vi "rsidr_core_global.vi"() -> ()   [LabVIEW 2020, in "Rohde&Schwarz CMWXP NR FR1 Measurement.lvlib"] (continued)
 "Rngtable Callback"="", "Coerce Callback"="", "Supported Models"="", "Instrument Options"="", "Check Status Callback"="", "Flags"=0, "Help"="Defines an upper limit for the carrier frequency error.\n\nAvailable Repeated Capabilities:\ninstance: i0, i1, i2, i3, i4, i5, i6, i7, i8, i9, i10, i11, i12, i13, i14, i15, i16, i17, i18, i19, i20, i21, i22, i23, i24, i25, i26, i27, i28, i29, i30, i31, i32\r\n\nRemote-control command(s):\nCONFigure:NRSub:MEAS<i>:PRACh:LIMit:FERRor"}, {"Level"=4, "Class Only"=FALSE, "Identifier"="RSCMWXPNRFR1M_ATTR_PRACH_LIMIT_FREQUENCY_ERROR_ENABLED", "Descriptive Name"="PRACH Limit Frequency Error Enabled", "Data Type"=enum."ViBoolean", "Command"="CONF:NRS:MEAS{instance}:PRAC:LIM:FERR", "Access"=enum."Read/Write", "Range Table"="", "Read Callback"="", "Write Callback"="", "Range Callback"="", "Check Callback"="", "Rngtable Callback"="", "Coerce Callback"="", "Supported Models"="", "Instrument Options"="", "Check Status Callback"="", "Flags"=0, "Help"="Enables or disables the limit check.\n\nAvailable Repeated Capabilities:\ninstance: i0, i1, i2, i3, i4, i5, i6, i7, i8, i9, i10, i11, i12, i13, i14, i15, i16, i17, i18, i19, i20, i21, i22, i23, i24, i25, i26, i27, i28, i29, i30, i31, i32\r\n\nRemote-control command(s):\nCONFigure:NRSub:MEAS<i>:PRACh:LIMit:FERRor"}, {"Level"=2, "Class Only"=TRUE, "Identifier"="", "Descriptive Name"="Results", "Data Type"=enum."ViInt32", "Command"="", "Access"=enum."Read Only", "Range Table"="", "Read Callback"="", "Write Callback"="", "Range Callback"="", "Check Callback"="", "Rngtable Callback"="", "Coerce Callback"="", "Supported Models"="", "Instrument Options"="", "Check Status Callback"="", "Flags"=0, "Help"="Results of the NR FR1 PRACH measurement"}, {"Level"=3, "Class Only"=TRUE, "Identifier"="", "Descriptive Name"="Detected Signal Configuration", "Data Type"=enum."ViInt32", "Command"="", "Access"=enum."Read Only", "Range Table"="", "Read Callback"="", "Write Callback"="", "Range Callback"="", "Check Callback"="", "Rngtable Callback"="", "Coerce Callback"="", "Supported Models"="", "Instrument Options"="", "Check Status Callback"="", "Flags"=0, "Help"="Returns the automatically detected or manually configured PRACH frequency offset for single-preamble measurements."}, {"Level"=4, "Class Only"=FALSE, "Identifier"="RSCMWXPNRFR1M_ATTR_FETCH_PRACH_FREQUENCY_OFFSET_RESULTS", "Descriptive Name"="Fetch PRACH Frequency Offset Results", "Data Type"=enum."RawString", "Command"="FETC:NRS:MEAS{instance}:PRAC:MOD:DPF?", "Access"=enum."Read Only", "Range Table"="", "Read Callback"="", "Write Callback"="", "Range Callback"="", "Check Callback"="", "Rngtable Callback"="", "Coerce Callback"="", "Supported Models"="", "Instrument Options"="", "Check Status Callback"="", "Flags"=0, "Help"="Returns the automatically detected or manually configured PRACH frequency offset for single-preamble measurements.\n\nAvailable Repeated Capabilities:\ninstance: i0, i1, i2, i3, i4, i5, i6, i7, i8, i9, i10, i11, i12, i13, i14, i15, i16, i17, i18, i19, i20, i21, i22, i23, i24, i25, i26, i27, i28, i29, i30, i31, i32\r\n\nRemote-control command(s):\nFETCh:NRSub:MEAS<i>:PRACh:MODulation:DPFoffset?"}, {"Level"=4, "Class Only"=FALSE, "Identifier"="RSCMWXPNRFR1M_ATTR_FETCH_PRACH_SEQUENCE_INDEX_RESULTS", "Descriptive Name"="Fetch PRACH Sequence Index Results", "Data Type"=enum."RawString", "Command"="FETC:NRS:MEAS{instance}:PRAC:MOD:DSIN?", "Access"=enum."Read Only", "Range Table"="", "Read Callback"="", "Write Callback"="", "Range Callback"="", "Check Callback"="", "Rngtable Callback"="", "Coerce Callback"="", "Supported Models"="", "Instrument Options"="", "Check Status Callback"="", "Flags"=0, "Help"="Returns the automatically detected or manually configured sequence index for single-preamble measurements.\n\nAvailable Repeated Capabilities:\ninstance: i0, i1, i2, i3, i4, i5, i6, i7, i8, i9, i10, i11, i12, i13, i14, i15, i16, i17, i18, i19, i20, i21, i22, i23, i24, i25, i26, i27, i28, i29, i30, i31, i32\r\n\nRemote-control command(s):\nFETCh:NRSub:MEAS<i>:PRACh:MODulation:DSINdex?"}, {"Level"=4, "Class Only"=FALSE, "Identifier"="RSCMWXPNRFR1M_ATTR_FETCH_PRACH_SEQUENCE_CORRELATION_RESULTS", "Descriptive Name"="Fetch PRACH Sequence Correlation Results", "Data Type"=enum."RawString", "Command"="FETC:NRS:MEAS{instance}:PRAC:MOD:SCOR?", "Access"=enum."Read Only", "Range Table"="", "Read Callback"="", "Write Callback"="", "Range Callback"="", "Check Callback"="", "Rngtable Callback"="", "Coerce Callback"="", "Supported Models"="", "Instrument Options"="", "Check Status Callback"="", "Flags"=0, "Help"="Returns the sequence correlation for single-preamble measurements. It indicates the correlation between the ideal preamble sequence determined from the parameter settings and the measured preamble sequence. A value of 1 corresponds to perfect correlation. A value much smaller than 1 indicates that the preamble sequence was not found.\n\nAvailable Repeated Capabilities:\ninstance: i0, i1, i2, i3, i4, i5, i6, i7, i8, i9, i10, i11, i12, i13, i14, i15, i16, i17, i18, i19, i20, i21, i22, i23, i24, i25, i26, i27, i28, i29, i30, i31, i32\r\n\nRemote-control command(s):\nFETCh:NRSub:MEAS<i>:PRACh:MODulation:SCORrelation?"}, {"Level"=4, "Class Only"=FALSE, "Identifier"="RSCMWXPNRFR1M_ATTR_FETCH_PRACH_FREQUENCY_OFFSET_PREAMBLE_RESULTS", "Descriptive Name"="Fetch PRACH Frequency Offset Preamble Results", "Data Type"=enum."RawString", "Command"="FETC:NRS:MEAS{instance}:PRAC:MOD:DPF:PRE{preamble}?", "Access"=enum."Read Only", "Range Table"="", "Read Callback"="", "Write Callback"="", "Range Callback"="", "Check Callback"="", "Rngtable Callback"="", "Coerce Callback"="", "Supported Models"="", "Instrument Options"="", "Check Status Callback"="", "Flags"=0, "Help"="Returns the automatically detected or manually configured PRACH frequency offset for a selected preamble of multi-preamble measurements.\n\nAvailable Repeated Capabilities:\ninstance: i0, i1, i2, i3, i4, i5, i6, i7, i8, i9, i10, i11, i12, i13, i14, i15, i16, i17, i18, i19, i20, i21, i22, i23, i24, i25, i26, i27, i28, i29, i30, i31, i32\r\npreamble: p1\r\n\nRemote-control command(s):\nFETCh:NRSub:MEAS<i>:PRACh:MODulation:DPFoffset:PREamble<Number>?"}, {"Level"=4, "Class Only"=FALSE, "Identifier"="RSCMWXPNRFR1M_ATTR_FETCH_PRACH_SEQUENCE_INDEX_PREAMBLE_RESULTS", "Descriptive Name"="Fetch PRACH Sequence Index Preamble Results", "Data Type"=enum."RawString", "Command"="FETC:NRS:MEAS{instance}:PRAC:MOD:DSIN:PRE{preamble}?", "Access"=enum."Read Only", "Range Table"="", "Read Callback"="", "Write Callback"="", "Range Callback"="", "Check Callback"="", "Rngtable Callback"="", "Coerce Callback"="", "Supported Models"="", "Instrument Options"="", "Check Status Callback"="", "Flags"=0, "Help"="Returns the automatically detected or manually configured sequence index for a selected preamble of multi-preamble measurements.\n\nAvailable Repeated Capabilities:\ninstance: i0, i1, i2, i3, i4, i5, i6, i7, i8, i9, i10, i11, i12, i13, i14, i15, i16, i17, i18, i19, i20, i21, i22, i23, i24, i25, i26, i27, i28, i29, i30, i31, i32\r\npreamble: p1\r\n\nRemote-control command(s):\nFETCh:NRSub:MEAS<i>:PRACh:MODulation:DSINdex:PREamble<Number>?"}, {"Level"=4, "Class Only"=FALSE, "Identifier"="RSCMWXPNRFR1M_ATTR_FETCH_PRACH_SEQUENCE_CORRELATION_PREAMBLE_RESULTS", "Descriptive Name"="Fetch PRACH Sequence Correlation Preamble Results", "Data Type"=enum."RawString", "Command"="FETC:NRS:MEAS{instance}:PRAC:MOD:SCOR:PRE{preamble}?", "Access"=enum."Read Only", "Range Table"="", "Read Callback"="", "Write Callback"="", "Range Callback"="", "Check Callback"="", "Rngtable Callback"="", "Coerce Callback"="", "Supported Models"="", "Instrument Options"="", "Check Status Callback"="", "Flags"=0, "Help"="Returns the sequence correlation for a selected preamble of multi-preamble measurements. It indicates the correlation between the ideal preamble sequence determined from the parameter settings and the measured preamble sequence. A value of 1 corresponds to perfect correlation. A value much smaller than 1 indicates that the preamble sequence was not found.\n\nAvailable Repeated Capabilities:\ninstance: i0, i1, i2, i3, i4, i5, i6, i7, i8, i9, i10, i11, i12, i13, i14, i15, i16, i17, i18, i19, i20, i21, i22, i23, i24, i25, i26, i27, i28, i29, i30, i31, i32\r\npreamble: p1\r\n\nRemote-control command(s):\nFETCh:NRSub:MEAS<i>:PRACh:MODulation:SCORrelation:PREamble<Number>?"}, {"Level"=3, "Class Only"=TRUE, "Identifier"="", "Descriptive Name"="Magnitude Error", "Data Type"=enum."ViInt32", "Command"="", "Access"=enum."Read Only", "Range Table"="", "Read Callback"="", "Write Callback"="", "Range Callback"="", "Check Callback"="", "Rngtable Callback"="", "Coerce Callback"="", "Supported Models"="", "Instrument Options"="", "Check Status Callback"="", "Flags"=0, "Help"="Returns the contents of the magnitude error vs subcarrier result diagram."}, {"Level"=4, "Class Only"=FALSE, "Identifier"="RSCMWXPNRFR1M_ATTR_READ_PRACH_MAGNITUDE_ERROR_CURRENT_TRACE_RESULTS", "Descriptive Name"="Read PRACH Magnitude Error Current Trace Results", "Data Type"=enum."RawString", "Command"="READ:NRS:MEAS{instance}:PRAC:TRAC:MERR:CURR?", "Access"=enum."Read Only", "Range Table"="", "Read Callback"="", "Write Callback"="", "Range Callback"="", "Check Callback"="", "Rngtable Callback"="", "Coerce Callback"="", "Supported Models"="", "Instrument Options"="", "Check Status Callback"="", "Flags"=0, "Help"="Starts a new single shot measurement and returns the values of the magnitude error traces. Each value is averaged over the samples in one preamble subcarrier. The results of the current traces can be retrieved.\n\nAvailable Repeated Capabilities:\ninstance: i0, i1, i2, i3, i4, i5, i6, i7, i8, i9, i10, i11, i12, i13, i14, i15, i16, i17, i18, i19, i20, i21, i22, i23, i24, i25, i26, i27, i28, i29, i30, i31, i32\r\n\nRemote-control command(s):\nREAD:NRSub:MEAS<i>:PRACh:TRACe:MERRor:CURRent?"}, {"Level"=4, "Class Only"=FALSE, "Identifier"="RSCMWXPNRFR1M_ATTR_READ_PRACH_MAGNITUDE_ERROR_AVERAGE_TRACE_RESULTS", "Descriptive Name"="Read PRACH Magnitude Error Average Trace Results", "Data Type"=enum."RawString", "Command"="READ:NRS:MEAS{instance}:PRAC:TRAC:MERR:AVER?", "Access"=enum."Read Only", "Range Table"="", "Read Callback"="", "Write Callback"="", "Range Callback"="", "Check Callback"="", "Rngtable Callback"="", "Coerce Callback"="", "Supported Models"="", "Instrument Options"="", "Check Status Callback"="", "Flags"=0, "Help"="Starts a new single shot measurement and returns the values of the magnitude error traces. Each value is averaged over the samples in one preamble subcarrier. The results of the average traces can be retrieved.\n\nAvailable Repeated Capabilities:\ninstance: i0, i1, i2, i3, i4, i5, i6, i7, i8, i9, i10, i11, i12, i13, i14, i15, i16, i17, i18, i19, i20, i21, i22, i23, i24, i25, i26, i27, i28, i29, i30, i31, i32\r\n\nRemote-control command(s):\nREAD:NRSub:MEAS<i>:PRACh:TRACe:MERRor:AVERage?"}, {"Level"=4, "Class Only"=FALSE, "Identifier"="RSCMWXPNRFR1M_ATTR_READ_PRACH_MAGNITUDE_ERROR_MAXIMUM_TRACE_RESULTS", "Descriptive Name"="Read PRACH Magnitude Error Maximum Trace Results", "Data Type"=enum."RawString", "Command"="READ:NRS:MEAS{instance}:PRAC:TRAC:MERR:MAX?", "Access"=enum."Read Only", "Range Table"="", "Read Callback"="", "Write Callback"="", "Range Callback"="", "Check Callback"="", "Rngtable Callback"="", "Coerce Callback"="", "Supported Models"="", "Instrument Options"="", "Check Status Callback"="", "Flags"=0, "Help"="Starts a new single shot measurement and returns the values of the magnitude error traces. Each value is averaged over the samples in one preamble subcarrier. The results of the maximum traces can be retrieved.\n\nAvailable Repeated Capabilities:\ninstance: i0, i1, i2, i3, i4, i5, i6, i7, i8, i9, i10, i11, i12, i13, i14, i15, i16, i17, i18, i19, i20, i21, i22, i23, i24, i25, i26, i27, i28, i29, i30, i31, i32\r\n\nRemote-control command(s):\nREAD:NRSub:MEAS<i>:PRACh:TRACe:MERRor:MAXimum?"}, {"Level"=4, "Class Only"=FALSE, "Identifier"="RSCMWXPNRFR1M_ATTR_FETCH_PRACH_MAGNITUDE_ERROR_CURRENT_TRACE_RESULTS", "Descriptive Name"="Fetch PRACH Magnitude Error Current Trace Results", "Data Type"=enum."RawString", "Command"="FETC:NRS:MEAS{instance}:PRAC:TRAC:MERR:CURR?", "Access"=enum."Read Only", "Range Table"="", "Read Callback"="", "Write Callback"="", "Range Callback"="", "Check Callback"="", "Rngtable Callback"="", "Coerce Callback"="", "Supported Models"="", "Instrument Options"="", "Check Status Callback"="", "Flags"=0, "Help"="Returns the values of the magnitude error traces. Each value is averaged over the samples in one preamble subcarrier. The results of the current traces can be retrieved.\n\nAvailable Repeated Capabilities:\ninstance: i0, i1, i2, i3, i4, i5, i6, i7, i8, i9, i10, i11, i12, i13, i14, i15, i16, i17, i18, i19, i20, i21, i22, i23, i24, i25, i26, i27, i28, i29, i30, i31, i32\r\n\nRemote-control command(s):\nFETCh:NRSub:MEAS<i>:PRACh:TRACe:MERRor:CURRent?"}, {"Level"=4, "Class Only"=FALSE, "Identifier"="RSCMWXPNRFR1M_ATTR_FETCH_PRACH_MAGNITUDE_ERROR_AVERAGE_TRACE_RESULTS", "Descriptive Name"="Fetch PRACH Magnitude Error Average Trace Results", "Data Type"=enum."RawString", "Command"="FETC:NRS:MEAS{instance}:PRAC:TRAC:MERR:AVER?", "Access"=enum."Read Only", "Range Table"="", "Read Callback"="", "Write Callback"="", "Range Callback"="", "Check Callback"="", "Rngtable Callback"="", "Coerce Callback"="", "Supported Models"="", "Instrument Options"="", "Check Status Callback"="", "Flags"=0, "Help"="Returns the values of the magnitude error traces. Each value is averaged over the samples in one preamble subcarrier. The results of the average traces can be retrieved.\n\nAvailable Repeated Capabilities:\ninstance: i0, i1, i2, i3, i4, i5, i6, i7, i8, i9, i10, i11, i12, i13, i14, i15, i16, i17, i18, i19, i20, i21, i22, i23, i24, i25, i26, i27, i28, i29, i30, i31, i32\r\n\nRemote-control command(s):\nFETCh:NRSub:MEAS<i>:PRACh:TRACe:MERRor:AVERage?"}, {"Level"=4, "Class Only"=FALSE, "Identifier"="RSCMWXPNRFR1M_ATTR_FETCH_PRACH_MAGNITUDE_ERROR_MAXIMUM_TRACE_RESULTS", "Descriptive Name"="Fetch PRACH Magnitude Error Maximum Trace Results", "Data Type"=enum."RawString", "Command"="FETC:NRS:MEAS{instance}:PRAC:TRAC:MERR:MAX?", "Access"=enum."Read Only", "Range Table"="", "Read Callback"="", "Write Callback"="", "Range Callback"="", "Check Callback"="", "Rngtable Callback"="", "Coerce Callback"="", "Supported Models"="", "Instrument Options"="", "Check Status Callback"="", "Flags"=0, "Help"="Returns the values of the magnitude error traces. Each value is averaged over the samples in one preamble subcarrier. The results of the maximum traces can be retrieved.\n\nAvailable Repeated Capabilities:\ninstance: i0, i1, i2, i3, i4, i5, i6, i7, i8, i9, i10, i11, i12, i13, i14, i15, i16, i17, i18, i19, i20, i21, i22, i23, i24, i25, i26, i27, i28, i29, i30, i31, i32\r\n\nRemote-control command(s):\nFETCh:NRSub:MEAS<i>:PRACh:TRACe:MERRor:MAXimum?"}, {"Level"=3, "Class Only"=TRUE, "Identifier"="", "Descriptive Name"="Phase Error", "Data Type"=enum."ViInt32", "Command"="", "Access"=enum."Read Only", "Range Table"="", "Read Callback"="", "Write Callback"="", "Range Callback"="", "Check Callback"="", "Rngtable Callback"="", "Coerce Callback"="", "Supported Models"="", "Instrument Options"="", "Check Status Callback"="", "Flags"=0, "Help"="Returns the contents of the phase error vs subcarrier result diagram."}, {"Level"=4, "Class Only"=FALSE, "Identifier"="RSCMWXPNRFR1M_ATTR_READ_PRACH_PHASE_ERROR_CURRENT_TRACE_RESULTS", "Descriptive Name"="Read PRACH Phase Error Current Trace Results", "Data Type"=enum."RawString", "Command"="READ:NRS:MEAS{instance}:PRAC:TRAC:PERR:CURR?", "Access"=enum."Read Only", "Range Table"="", "Read Callback"="", "Write Callback"="", "Range Callback"="", "Check Callback"="", "Rngtable Callback"="", "Coerce Callback"="", "Supported Models"="", "Instrument Options"="", "Check Status Callback"="", "Flags"=0, "Help"="Starts a new single shot measurement and returns the values of the phase error traces. Each value is averaged over the samples in one preamble subcarrier. The results of the current traces can be retrieved.\n\nAvailable Repeated Capabilities:\ninstance: i0, i1, i2, i3, i4, i5, i6, i7, i8, i9, i10, i11, i12, i13, i14, i15, i16, i17, i18, i19, i20, i21, i22, i23, i24, i25, i26, i27, i28, i29, i30, i31, i32\r\n\nRemote-control command(s):\nREAD:NRSub:MEAS<i>:PRACh:TRACe:PERRor:CURRent?"}, {"Level"=4, "Class Only"=FALSE, "Identifier"="RSCMWXPNRFR1M_ATTR_READ_PRACH_PHASE_ERROR_AVERAGE_TRACE_RESULTS", "Descriptive Name"="Read PRACH Phase Error Average Trace Results", "Data Type"=enum."RawString", "Command"="READ:NRS:MEAS{instance}:PRAC:TRAC:PERR:AVER?", "Access"=enum."Read Only", "Range Table"="", "Read Callback"="", "Write Callback"="", "Range Callback"="", "Check Callback"="", "Rngtable Callback"="", "Coerce Callback"="", "Supported Models"="", "Instrument Options"="", "Check Status Callback"="", "Flags"=0, "Help"="Starts a new single shot measurement and returns the values of the phase error traces. Each value is averaged over the samples in one preamble subcarrier. The results of the average traces can be retrieved.\n\nAvailable Repeated Capabilities:\ninstance: i0, i1, i2, i3, i4, i5, i6, i7, i8, i9, i10, i11, i12, i13, i14, i15, i16, i17, i18, i19, i20, i21, i22, i23, i24, i25, i26, i27, i28, i29, i30, i31, i32\r\n\nRemote-control command(s):\nREAD:NRSub:MEAS<i>:PRACh:TRACe:PERRor:AVERage?"}, {"Level"=4, "Class Only"=FALSE, "Identifier"="RSCMWXPNRFR1M_ATTR_READ_PRACH_PHASE_ERROR_MAXIMUM_TRACE_RESULTS", "Descriptive Name"="Read PRACH Phase Error Maximum Trace Results", "Data Type"=enum."RawString", "Command"="READ:NRS:MEAS{instance}:PRAC:TRAC:PERR:MAX?", "Access"=enum."Read Only", "Range Table"="", "Read Callback"="", "Write Callback"="", "Range Callback"="", "Check Callback"="", "Rngtable Callback"="", "Coerce Callback"="", "Supported Models"="", "Instrument Options"="", "Check Status Callback"="", "Flags"=0, "Help"="Starts a new single shot measurement and returns the values of the phase error traces. Each value is averaged over the samples in one preamble subcarrier. The results of the maximum traces can be retrieved.\n\nAvailable Repeated Capabilities:\ninstance: i0, i1, i2, i3, i4, i5, i6, i7, i8, i9, i10, i11, i12, i13, i14, i15, i16, i17, i18, i19, i20, i21, i22, i23, i24, i25, i26, i27, i28, i29, i30, i31, i32\r\n\nRemote-control command(s):\nREAD:NRSub:MEAS<i>:PRACh:TRACe:PERRor:MAXimum?"}, {"Level"=4, "Class Only"=FALSE, "Identifier"="RSCMWXPNRFR1M_ATTR_FETCH_PRACH_PHASE_ERROR_CURRENT_TRACE_RESULTS", "Descriptive Name"="Fetch PRACH Phase Error Current Trace Results", "Data Type"=enum."RawString", "Command"="FETC:NRS:MEAS{instance}:PRAC:TRAC:PERR:CURR?", "Access"=enum."Read Only", "Range Table"="", "Read Callback"="", "Write Callback"="", "Range Callback"="", "Check Callback"="", "Rngtable Callback"="", "Coerce Callback"="", "Supported Models"="", "Instrument Options"="", "Check Status Callback"="", "Flags"=0, "Help"="Returns the values of the phase error traces. Each value is averaged over the samples in one preamble subcarrier. The results of the current traces can be retrieved.\n\nAvailable Repeated Capabilities:\ninstance: i0, i1, i2, i3, i4, i5, i6, i7, i8, i9, i10, i11, i12, i13, i14, i15, i16, i17, i18, i19, i20, i21, i22, i23, i24, i25, i26, i27, i28, i29, i30, i31, i32\r\n\nRemote-control command(s):\nFETCh:NRSub:MEAS<i>:PRACh:TRACe:PERRor:CURRent?"}, {"Level"=4, "Class Only"=FALSE, "Identifier"="RSCMWXPNRFR1M_ATTR_FETCH_PRACH_PHASE_ERROR_AVERAGE_TRACE_RESULTS", "Descriptive Name"="Fetch PRACH Phase Error Average Trace Results", "Data Type"=enum."RawString", "Command"="FETC:NRS:MEAS{instance}:PRAC:TRAC:PERR:AVER?", "Access"=enum."Read Only", "Range Table"="", "Read Callback"="", "Write Callback"="", "Range Callback"="", "Check Callback"="", "Rngtable Callback"="", "Coerce Callback"="", "Supported Models"="", "Instrument Options"="", "Check Status Callback"="", "Flags"=0, "Help"="Returns the values of the phase error traces. Each value is averaged over the samples in one preamble subcarrier. The results of the average traces can be retrieved.\n\nAvailable Repeated Capabilities:\ninstance: i0, i1, i2, i3, i4, i5, i6, i7, i8, i9, i10, i11, i12, i13, i14, i15, i16, i17, i18, i19, i20, i21, i22, i23, i24, i25, i26, i27, i28, i29, i30, i31, i32\r\n\nRemote-control command(s):\nFETCh:NRSub:MEAS<i>:PRACh:TRACe:PERRor:AVERage?"}, {"Level"=4, "Class Only"=FALSE, "Identifier"="RSCMWXPNRFR1M_ATTR_FETCH_PRACH_PHASE_ERROR_MAXIMUM_TRACE_RESULTS", "Descriptive Name"="Fetch PRACH Phase Error Maximum Trace Results", "Data Type"=enum."RawString", "Command"="FETC:NRS:MEAS{instance}:PRAC:TRAC:PERR:MAX?", "Access"=enum."Read Only", "Range Table"="", "Read Callback"="", "Write Callback"="", "Range Callback"="", "Check Callback"="", "Rngtable Callback"="", "Coerce Callback"="", "Supported Models"="", "Instrument Options"="", "Check Status Callback"="", "Flags"=0, "Help"="Returns the values of the phase error traces. Each value is averaged over the samples in one preamble subcarrier. The results of the maximum traces can be retrieved.\n\nAvailable Repeated Capabilities:\ninstance: i0, i1, i2, i3, i4, i5, i6, i7, i8, i9, i10, i11, i12, i13, i14, i15, i16, i17, i18, i19, i20, i21, i22, i23, i24, i25, i26, i27, i28, i29, i30, i31, i32\r\n\nRemote-control command(s):\nFETCh:NRSub:MEAS<i>:PRACh:TRACe:PERRor:MAXimum?"}, {"Level"=3, "Class Only"=TRUE, "Identifier"="", "Descriptive Name"="EVM vs Subcarrier", "Data Type"=enum."ViInt32", "Command"="", "Access"=enum."Read Only", "Range Table"="", "Read Callback"="", "Write Callback"="", "Range Callback"="", "Check Callback"="", "Rngtable Callback"="", "Coerce Callback"="", "Supported Models"="", "Instrument Options"="", "Check Status Callback"="", "Flags"=0, "Help"="Returns the contents of the EVM vs subcarrier result diagram."}, {"Level"=4, "Class Only"=FALSE, "Identifier"="RSCMWXPNRFR1M_ATTR_READ_PRACH_EVM_VS_SUBCARRIER_CURRENT_TRACE_RESULTS", "Descriptive Name"="Read PRACH EVM Vs Subcarrier Current Trace Results", "Data Type"=enum."RawString", "Command"="READ:NRS:MEAS{instance}:PRAC:TRAC:EVM:CURR?", "Access"=enum."Read Only", "Range Table"="", "Read Callback"="", "Write Callback"="", "Range Callback"="", "Check Callback"="", "Rngtable Callback"="", "Coerce Callback"="", "Supported Models"="", "Instrument Options"="", "Check Status Callback"="", "Flags"=0, "Help"="Starts a new single shot measurement and returns the values of the EVM vs subcarrier traces. Each value is averaged over the samples in one preamble subcarrier. The results of the current traces can be retrieved.\n\nAvailable Repeated Capabilities:\ninstance: i0, i1, i2, i3, i4, i5, i6, i7, i8, i9, i10, i11, i12, i13, i14, i15, i16, i17, i18, i19, i20, i21, i22, i23, i24, i25, i26, i27, i28, i29, i30, i31, i32\r\n\nRemote-control command(s):\nREAD:NRSub:MEAS<i>:PRACh:TRACe:EVM:CURRent?"}, {"Level"=4, "Class Only"=FALSE, "Identifier"="RSCMWXPNRFR1M_ATTR_READ_PRACH_EVM_VS_SUBCARRIER_AVERAGE_TRACE_RESULTS", "Descriptive Name"="Read PRACH EVM Vs Subcarrier Average Trace Results", "Data Type"=enum."RawString", "Command"="READ:NRS:MEAS{instance}:PRAC:TRAC:EVM:AVER?", "Access"=enum."Read Only", "Range Table"="", "Read Callback"="", "Write Callback"="", "Range Callback"="", "Check Callback"="", "Rngtable Callback"="", "Coerce Callback"="", "Supported Models"="", "Instrument Options"="", "Check Status Callback"="", "Flags"=0, "Help"="Starts a new single shot measurement and returns the values of the EVM vs subcarrier traces. Each value is averaged over the samples in one preamble subcarrier. The results of the average traces can be retrieved.\n\nAvailable Repeated Capabilities:\ninstance: i0, i1, i2, i3, i4, i5, i6, i7, i8, i9, i10, i11, i12, i13, i14, i15, i16, i17, i18, i19, i20, i21, i22, i23, i24, i25, i26, i27, i28, i29, i30, i31, i32\r\n\nRemote-control command(s):\nREAD:NRSub:MEAS<i>:PRACh:TRACe:EVM:AVERage?"}, {"Level"=4, "Class Only"=FALSE, "Identifier"="RSCMWXPNRFR1M_ATTR_READ_PRACH_EVM_VS_SUBCARRIER_MAXIMUM_TRACE_RESULTS", "Descriptive Name"="Read PRACH EVM Vs Subcarrier Maximum Trace Results", "Data Type"=enum."RawString", "Command"="READ:NRS:MEAS{instance}:PRAC:TRAC:EVM:MAX?", "Access"=enum."Read Only", "Range Table"="", "Read Callback"="", "Write Callback"="", "Range Callback"="", "Check Callback"="", "Rngtable Callback"="", "Coerce Callback"="", "Supported Models"="", "Instrument Options"="", "Check Status Callback"="", "Flags"=0, "Help"="Starts a new single shot measurement and returns the values of the EVM vs subcarrier traces. Each value is averaged over the samples in one preamble subcarrier. The results of the maximum traces can be retrieved.\n\nAvailable Repeated Capabilities:\ninstance: i0, i1, i2, i3, i4, i5, i6, i7, i8, i9, i10, i11, i12, i13, i14, i15, i16, i17, i18, i19, i20, i21, i22, i23, i24, i25, i26, i27, i28, i29, i30, i31, i32\r\n\nRemote-control command(s):\nREAD:NRSub:MEAS<i>:PRACh:TRACe:EVM:MAXimum?"}, {"Level"=4, "Class Only"=FALSE, "Identifier"="RSCMWXPNRFR1M_ATTR_FETCH_PRACH_EVM_VS_SUBCARRIER_CURRENT_TRACE_RESULTS", "Descriptive Name"="Fetch PRACH EVM Vs Subcarrier Current Trace Results", "Data Type"=enum."RawString", "Command"="FETC:NRS:MEAS{instance}:PRAC:TRAC:EVM:CURR?", "Access"=enum."Read Only", "Range Table"="", "Read Callback"="", "Write Callback"="", "Range Callback"="", "Check Callback"="", "Rngtable Callback"="", "Coerce Callback"="", "Supported Models"="", "Instrument Options"="", "Check Status Callback"="", "Flags"=0, "Help"="Returns the values of the EVM vs subcarrier traces. Each value is averaged over the samples in one preamble subcarrier. The results of the current traces can be retrieved.\n\nAvailable Repeated Capabilities:\ninstance: i0, i1, i2, i3, i4, i5, i6, i7, i8, i9, i10, i11, i12, i13, i14, i15, i16, i17, i18, i19, i20, i21, i22, i23, i24, i25, i26, i27, i28, i29, i30, i31, i32\r\n\nRemote-control command(s):\nFETCh:NRSub:MEAS<i>:PRACh:TRACe:EVM:CURRent?"}, {"Level"=4, "Class Only"=FALSE, "Identifier"="RSCMWXPNRFR1M_ATTR_FETCH_PRACH_EVM_VS_SUBCARRIER_AVERAGE_TRACE_RESULTS", "Descriptive Name"="Fetch PRACH EVM Vs Subcarrier Average Trace Results", "Data Type"=enum."RawString", "Command"="FETC:NRS:MEAS{instance}:PRAC:TRAC:EVM:AVER?", "Access"=enum."Read Only", "Range Table"="", "Read Callback"="", "Write Callback"="", "Range Callback"="", "Check Callback"="", "Rngtable Callback"="", "Coerce Callback"="", "Supported Models"="", "Instrument Options"="", "Check Status Callback"="", "Flags"=0, "Help"="Returns the values of the EVM vs subcarrier traces. Each value is averaged over the samples in one preamble subcarrier. The results of the average traces can be retrieved.\n\nAvailable Repeated Capabilities:\ninstance: i0, i1, i2, i3, i4, i5, i6, i7, i8, i9, i10, i11, i12, i13, i14, i15, i16, i17, i18, i19, i20, i21, i22, i23, i24, i25, i26, i27, i28, i29, i30, i31, i32\r\n\nRemote-control command(s):\nFETCh:NRSub:MEAS<i>:PRACh:TRACe:EVM:AVERage?"}, {"Level"=4, "Class Only"=FALSE, "Identifier"="RSCMWXPNRFR1M_ATTR_FETCH_PRACH_EVM_VS_SUBCARRIER_MAXIMUM_TRACE_RESULTS", "Descriptive Name"="Fetch PRACH EVM Vs Subcarrier Maximum Trace Results", "Data Type"=enum."RawString", "Command"="FETC:NRS:MEAS{instance}:PRAC:TRAC:EVM:MAX?", "Access"=enum."Read Only", "Range Table"="", "Read Callback"="", "Write Callback"="", "Range Callback"="", "Check Callback"="", "Rngtable Callback"="", "Coerce Callback"="", "Supported Models"="", "Instrument Options"="", "Check Status Callback"="", "Flags"=0, "Help"="Returns the values of the EVM vs subcarrier traces. Each value is averaged over the samples in one preamble subcarrier. The results of the maximum traces can be retrieved.\n\nAvailable Repeated Capabilities:\ninstance: i0, i1, i2, i3, i4, i5, i6, i7, i8, i9, i10, i11, i12, i13, i14, i15, i16, i17, i18, i19, i20, i21, i22, i23, i24, i25, i26, i27, i28, i29, i30, i31, i32\r\n\nRemote-control command(s):\nFETCh:NRSub:MEAS<i>:PRACh:TRACe:EVM:MAXimum?"}, {"Level"=3, "Class Only"=TRUE, "Identifier"="", "Descriptive Name"="EVM vs Preamble", "Data Type"=enum."ViInt32", "Command"="", "Access"=enum."Read Only", "Range Table"="", "Read Callback"="", "Write Callback"="", "Range Callback"="", "Check Callback"="", "Rngtable Callback"="", "Coerce Callback"="", "Supported Models"="", "Instrument Options"="", "Check Status Callback"="", "Flags"=0, "Help"="Returns the contents of the EVM vs preamble result diagram."}, {"Level"=4, "Class Only"=FALSE, "Identifier"="RSCMWXPNRFR1M_ATTR_READ_PRACH_EVM_VS_PREAMBLE_TRACE_RESULTS", "Descriptive Name"="Read PRACH EVM Vs Preamble Trace Results", "Data Type"=enum."RawString", "Command"="READ:NRS:MEAS{instance}:PRAC:TRAC:EVPR?", "Access"=enum."Read Only", "Range Table"="", "Read Callback"="", "Write Callback"="", "Range Callback"="", "Check Callback"="", "Rngtable Callback"="", "Coerce Callback"="", "Supported Models"="", "Instrument Options"="", "Check Status Callback"="", "Flags"=0, "Help"="Starts a new single shot measurement and returns the values of the EVM vs preamble traces.\n\nAvailable Repeated Capabilities:\ninstance: i0, i1, i2, i3, i4, i5, i6, i7, i8, i9, i10, i11, i12, i13, i14, i15, i16, i17, i18, i19, i20, i21, i22, i23, i24, i25, i26, i27, i28, i29, i30, i31, i32\r\n\nRemote-control command(s):\nREAD:NRSub:MEAS<i>:PRACh:TRACe:EVPReamble?"}, {"Level"=4, "Class Only"=FALSE, "Identifier"="RSCMWXPNRFR1M_ATTR_FETCH_PRACH_EVM_VS_PREAMBLE_TRACE_RESULTS", "Descriptive Name"="Fetch PRACH EVM Vs Preamble Trace Results", "Data Type"=enum."RawString", "Command"="FETC:NRS:MEAS{instance}:PRAC:TRAC:EVPR?", "Access"=enum."Read Only", "Range Table"="", "Read Callback"="", "Write Callback"="", "Range Callback"="", "Check Callback"="", "Rngtable Callback"="", "Coerce Callback"="", "Supported Models"="", "Instrument Options"="", "Check Status Callback"="", "Flags"=0, "Help"="Returns the values of the EVM vs preamble traces.\n\nAvailable Repeated Capabilities:\ninstance: i0, i1, i2, i3, i4, i5, i6, i7, i8, i9, i10, i11, i12, i13, i14, i15, i16, i17, i18, i19, i20, i21, i22, i23, i24, i25, i26, i27, i28, i29, i30, i31, i32\r\n\nRemote-control command(s):\nFETCh:NRSub:MEAS<i>:PRACh:TRACe:EVPReamble?"}, {"Level"=3, "Class Only"=TRUE, "Identifier"="", "Descriptive Name"="Power vs Preamble", "Data Type"=enum."ViInt32", "Command"="", "Access"=enum."Read Only", "Range Table"="", "Read Callback"="", "Write Callback"="", "Range Callback"="", "Check Callback"="", "Rngtable Callback"="", "Coerce Callback"="", "Supported Models"="", "Instrument Options"="", "Check Status Callback"="", "Flags"=0, "Help"="Returns the contents of the power vs preamble result diagram."}, {"Level"=4, "Class Only"=FALSE, "Identifier"="RSCMWXPNRFR1M_ATTR_READ_PRACH_POWER_VS_PREAMBLE_TRACE_RESULTS", "Descriptive Name"="Read PRACH Power Vs Preamble Trace Results", "Data Type"=enum."RawString", "Command"="READ:NRS:MEAS{instance}:PRAC:TRAC:PVPR?", "Access"=enum."Read Only", "Range Table"="", "Read Callback"="", "Write Callback"="", "Range Callback"="", "Check Callback"="", "Rngtable Callback"="", "Coerce Callback"="", "Supported Models"="", "Instrument Options"="", "Check Status Callback"="", "Flags"=0, "Help"="Starts a new single shot measurement and returns the values of the power vs preamble traces.\n\nAvailable Repeated Capabilities:\ninstance: i0, i1, i2, i3, i4, i5, i6, i7, i8, i9, i10, i11, i12, i13, i14, i15, i16, i17, i18, i19, i20, i21, i22, i23, i24, i25, i26, i27, i28, i29, i30, i31, i32\r\n\nRemote-control command(s):\nREAD:NRSub:MEAS<i>:PRACh:TRACe:PVPReamble?"}, {"Level"=4, "Class Only"=FALSE, "Identifier"="RSCMWXPNRFR1M_ATTR_FETCH_PRACH_POWER_VS_PREAMBLE_TRACE_RESULTS", "Descriptive Name"="Fetch PRACH Power Vs Preamble Trace Results", "Data Type"=enum."RawString", "Command"="FETC:NRS:MEAS{instance}:PRAC:TRAC:PVPR?", "Access"=enum."Read Only", "Range Table"="", "Read Callback"="", "Write Callback"="", "Range Callback"="", "Check Callback"="", "Rngtable Callback"="", "Coerce Callback"="", "Supported Models"="", "Instrument Options"="", "Check Status Callback"="", "Flags"=0, "Help"="Returns the values of the power vs preamble traces.\n\nAvailable Repeated Capabilities:\ninstance: i0, i1, i2, i3, i4, i5, i6, i7, i8, i9, i10, i11, i12, i13, i14, i15, i16, i17, i18, i19, i20, i21, i22, i23, i24, i25, i26, i27, i28, i29, i30, i31, i32\r\n\nRemote-control command(s):\nFETCh:NRSub:MEAS<i>:PRACh:TRACe:PVPReamble?"}, {"Level"=3, "Class Only"=TRUE, "Identifier"="", "Descriptive Name"="IQ Constellation", "Data Type"=enum."ViInt32", "Command"="", "Access"=enum."Read Only", "Range Table"="", "Read Callback"="", "Write Callback"="", "Range Callback"="", "Check Callback"="", "Rngtable Callback"="", "Coerce Callback"="", "Supported Models"="", "Instrument Options"="", "Check Status Callback"="", "Flags"=0, "Help"="The following attributes return the contents of the I/Q constellation diagram."}, {"Level"=4, "Class Only"=FALSE, "Identifier"="RSCMWXPNRFR1M_ATTR_FETCH_PRACH_IQ_CONSTELLATION_TRACE_RESULTS", "Descriptive Name"="Fetch PRACH IQ Constellation Trace Results", "Data Type"=enum."RawString", "Command"="FETC:NRS:MEAS{instance}:PRAC:TRAC:IQ?", "Access"=enum."Read Only", "Range Table"="", "Read Callback"="", "Write Callback"="", "Range Callback"="", "Check Callback"="", "Rngtable Callback"="", "Coerce Callback"="", "Supported Models"="", "Instrument Options"="", "Check Status Callback"="", "Flags"=0, "Help"="Returns the results in the I/Q constellation diagram. There is one pair of values per modulation symbol. The number of modulation symbols equals the number of subcarriers and depends on the preamble format. The results are returned in the following order: <Reliability>, {<IPhase>, <QPhase>}symbol 1, ..., {<IPhase>, <QPhase>}symbol n\n\nAvailable Repeated Capabilities:\ninstance: i0, i1, i2, i3, i4, i5, i6, i7, i8, i9, i10, i11, i12, i13, i14, i15, i16, i17, i18, i19, i20, i21, i22, i23, i24, i25, i26, i27, i28, i29, i30, i31, i32\r\n\nRemote-control command(s):\nFETCh:NRSub:MEAS<i>:PRACh:TRACe:IQ?"}, {"Level"=3, "Class Only"=TRUE, "Identifier"="", "Descriptive Name"="Power Dynamics", "Data Type"=enum."ViInt32", "Command"="", "Access"=enum."Read Only", "Range Table"="", "Read Callback"="", "Write Callback"="", "Range Callback"="", "Check Callback"="", "Rngtable Callback"="", "Coerce Callback"="", "Supported Models"="", "Instrument Options"="", "Check Status Callback"="", "Flags"=0, "Help"="Returns the contents of the power dynamics result diagram."}, {"Level"=4, "Class Only"=FALSE, "Identifier"="RSCMWXPNRFR1M_ATTR_READ_PRACH_POWER_DYNAMICS_CURRENT_TRACE_RESULTS", "Descriptive Name"="Read PRACH Power Dynamics Current Trace Results", "Data Type"=enum."RawString", "Command"="READ:NRS:MEAS{instance}:PRAC:TRAC:PDYN:CURR?", "Access"=enum."Read Only", "Range Table"="", "Read Callback"="", "Write Callback"="", "Range Callback"="", "Check Callback"="", "Rngtable Callback"="", "Coerce Callback"="", "Supported Models"="", "Instrument Options"="", "Check Status Callback"="", "Flags"=0, "Help"="Starts a new single shot measurement and returns the values of the power dynamics traces. Each value is sampled with 48 Ts, corresponding to 1.5625 us. The results of the current traces can be retrieved.\n\nAvailable Repeated Capabilities:\ninstance: i0, i1, i2, i3, i4, i5, i6, i7, i8, i9, i10, i11, i12, i13, i14, i15, i16, i17, i18, i19, i20, i21, i22, i23, i24, i25, i26, i27, i28, i29, i30, i31, i32\r\n\nRemote-control command(s):\nREAD:NRSub:MEAS<i>:PRACh:TRACe:PDYNamics:CURRent?"}, {"Level"=4, "Class Only"=FALSE, "Identifier"="RSCMWXPNRFR1M_ATTR_READ_PRACH_POWER_DYNAMICS_AVERAGE_TRACE_RESULTS", "Descriptive Name"="Read PRACH Power Dynamics Average Trace Results", "Data Type"=enum."RawString", "Command"="READ:NRS:MEAS{instance}:PRAC:TRAC:PDYN:AVER?", "Access"=enum."Read Only", "Range Table"="", "Read Callback"="", "Write Callback"="", "Range Callback"="", "Check Callback"="", "Rngtable Callback"="", "Coerce Callback"="", "Supported Models"="", "Instrument Options"="", "Check Status Callback"="", "Flags"=0, "Help"="Starts a new single shot measurement and returns the values of the power dynamics traces. Each value is sampled with 48 Ts, corresponding to 1.5625 us. The results of the average traces can be retrieved.\n\nAvailable Repeated Capabilities:\ninstance: i0, i1, i2, i3, i4, i5, i6, i7, i8, i9, i10, i11, i12, i13, i14, i15, i16, i17, i18, i19, i20, i21, i22, i23, i24, i25, i26, i27, i28, i29, i30, i31, i32\r\n\nRemote-control command(s):\nREAD:NRSub:MEAS<i>:PRACh:TRACe:PDYNamics:AVERage?"}, {"Level"=4, "Class Only"=FALSE, "Identifier"="RSCMWXPNRFR1M_ATTR_READ_PRACH_POWER_DYNAMICS_MAXIMUM_TRACE_RESULTS", "Descriptive Name"="Read PRACH Power Dynamics Maximum Trace Results", "Data Type"=enum."RawString", "Command"="READ:NRS:MEAS{instance}:PRAC:TRAC:PDYN:MAX?", "Access"=enum."Read Only", "Range Table"="", "Read Callback"="", "Write Callback"="", "Range Callback"="", "Check Callback"="", "Rngtable Callback"="", "Coerce Callback"="", "Supported Models"="", "Instrument Options"="", "Check Status Callback"="", "Flags"=0, "Help"="Starts a new single shot measurement and returns the values of the power dynamics traces. Each value is sampled with 48 Ts, corresponding to 1.5625 us. The results of the maximum traces can be retrieved.\n\nAvailable Repeated Capabilities:\ninstance: i0, i1, i2, i3, i4, i5, i6, i7, i8, i9, i10, i11, i12, i13, i14, i15, i16, i17, i18, i19, i20, i21, i22, i23, i24, i25, i26, i27, i28, i29, i30, i31, i32\r\n\nRemote-control command(s):\nREAD:NRSub:MEAS<i>:PRACh:TRACe:PDYNamics:MAXimum?"}, {"Level"=4, "Class Only"=FALSE, "Identifier"="RSCMWXPNRFR1M_ATTR_FETCH_PRACH_POWER_DYNAMICS_CURRENT_TRACE_RESULTS", "Descriptive Name"="Fetch PRACH Power Dynamics Current Trace Results", "Data Type"=enum."RawString", "Command"="FETC:NRS:MEAS{instance}:PRAC:TRAC:PDYN:CURR?", "Access"=enum."Read Only", "Range Table"="", "Read Callback"="", "Write Callback"="", "Range Callback"="", "Check Callback"="", "Rngtable Callback"="", "Coerce Callback"="", "Supported Models"="", "Instrument Options"="", "Check Status Callback"="", "Flags"=0, "Help"="Returns the values of the power dynamics traces. Each value is sampled with 48 Ts, corresponding to 1.5625 us. The results of the current traces can be retrieved.\n\nAvailable Repeated Capabilities:\ninstance: i0, i1, i2, i3, i4, i5, i6, i7, i8, i9, i10, i11, i12, i13, i14, i15, i16, i17, i18, i19, i20, i21, i22, i23, i24, i25, i26, i27, i28, i29, i30, i31, i32\r\n\nRemote-control command(s):\nFETCh:NRSub:MEAS<i>:PRACh:TRACe:PDYNamics:CURRent?"}, {"Level"=4, "Class Only"=FALSE, "Identifier"="RSCMWXPNRFR1M_ATTR_FETCH_PRACH_POWER_DYNAMICS_AVERAGE_TRACE_RESULTS", "Descriptive Name"="Fetch PRACH Power Dynamics Average Trace Results", "Data Type"=enum."RawString", "Command"="FETC:NRS:MEAS{instance}:PRAC:TRAC:PDYN:AVER?", "Access"=enum."Read Only", "Range Table"="", "Read Callback"="", "Write Callback"="", "Range Callback"="", "Check Callback"="", "Rngtable Callback"="", "Coerce Callback"="", "Supported Models"="", "Instrument Options"="", "Check Status Callback"="", "Flags"=0, "Help"="Returns the values of the power dynamics traces. Each value is sampled with 48 Ts, corresponding to 1.5625 us. The results of the average traces can be retrieved.\n\nAvailable Repeated Capabilities:\ninstance: i0, i1, i2, i3, i4, i5, i6, i7, i8, i9, i10, i11, i12, i13, i14, i15, i16, i17, i18, i19, i20, i21, i22, i23, i24, i25, i26, i27, i28, i29, i30, i31, i32\r\n\nRemote-control command(s):\nFETCh:NRSub:MEAS<i>:PRACh:TRACe:PDYNamics:AVERage?"}, {"Level"=4, "Class Only"=FALSE, "Identifier"="RSCMWXPNRFR1M_ATTR_FETCH_PRACH_POWER_DYNAMICS_MAXIMUM_TRACE_RESULTS", "Descriptive Name"="Fetch PRACH Power Dynamics Maximum Trace Results", "Data Type"=enum."RawString", "Command"="FETC:NRS:MEAS{instance}:PRAC:TRAC:PDYN:MAX?", 
